vi "update fuel array.vi"(8 "Decrement fuel?":bool, 9 "Game Parameters":T3, 10 "step count":i32, 11 "Arrays and values":T1={"Score Array"=[], "Lowest high score"=0.0, "Score"=0.0, "Ceiling"=0.0, "Floor"=0.0, "Ceiling Array"=[], "Floor array"=[], "Helicopter height"=0.0, "Helicopter array"=[], "Fuel"=0.0, "Fuel array"=[], "fuel counter"=0, "obstacle counter"=0, "Obstacle array"=[], "helicopter v_0"=0.0, "helicopter a_0"=0.0, "Obstacle height"=300.0}) -> (2 "Fuel (L)":dbl(knob)=150.0 scale=0.0..300.0, 3 "Arrays and Heights":T1={"Score Array"=[], "Lowest high score"=0.0, "Score"=0.0, "Ceiling"=0.0, "Floor"=0.0, "Ceiling Array"=[], "Floor array"=[], "Helicopter height"=0.0, "Helicopter array"=[], "Fuel"=300.0, "Fuel array"=[], "fuel counter"=0, "obstacle counter"=0, "Obstacle array"=[], "helicopter v_0"=0.0, "helicopter a_0"=0.0, "Obstacle height"=300.0})   [LabVIEW 2017]
uses:
  controls/arrays and heights.ctl
  controls/scores.ctl
  controls/game parameters.ctl
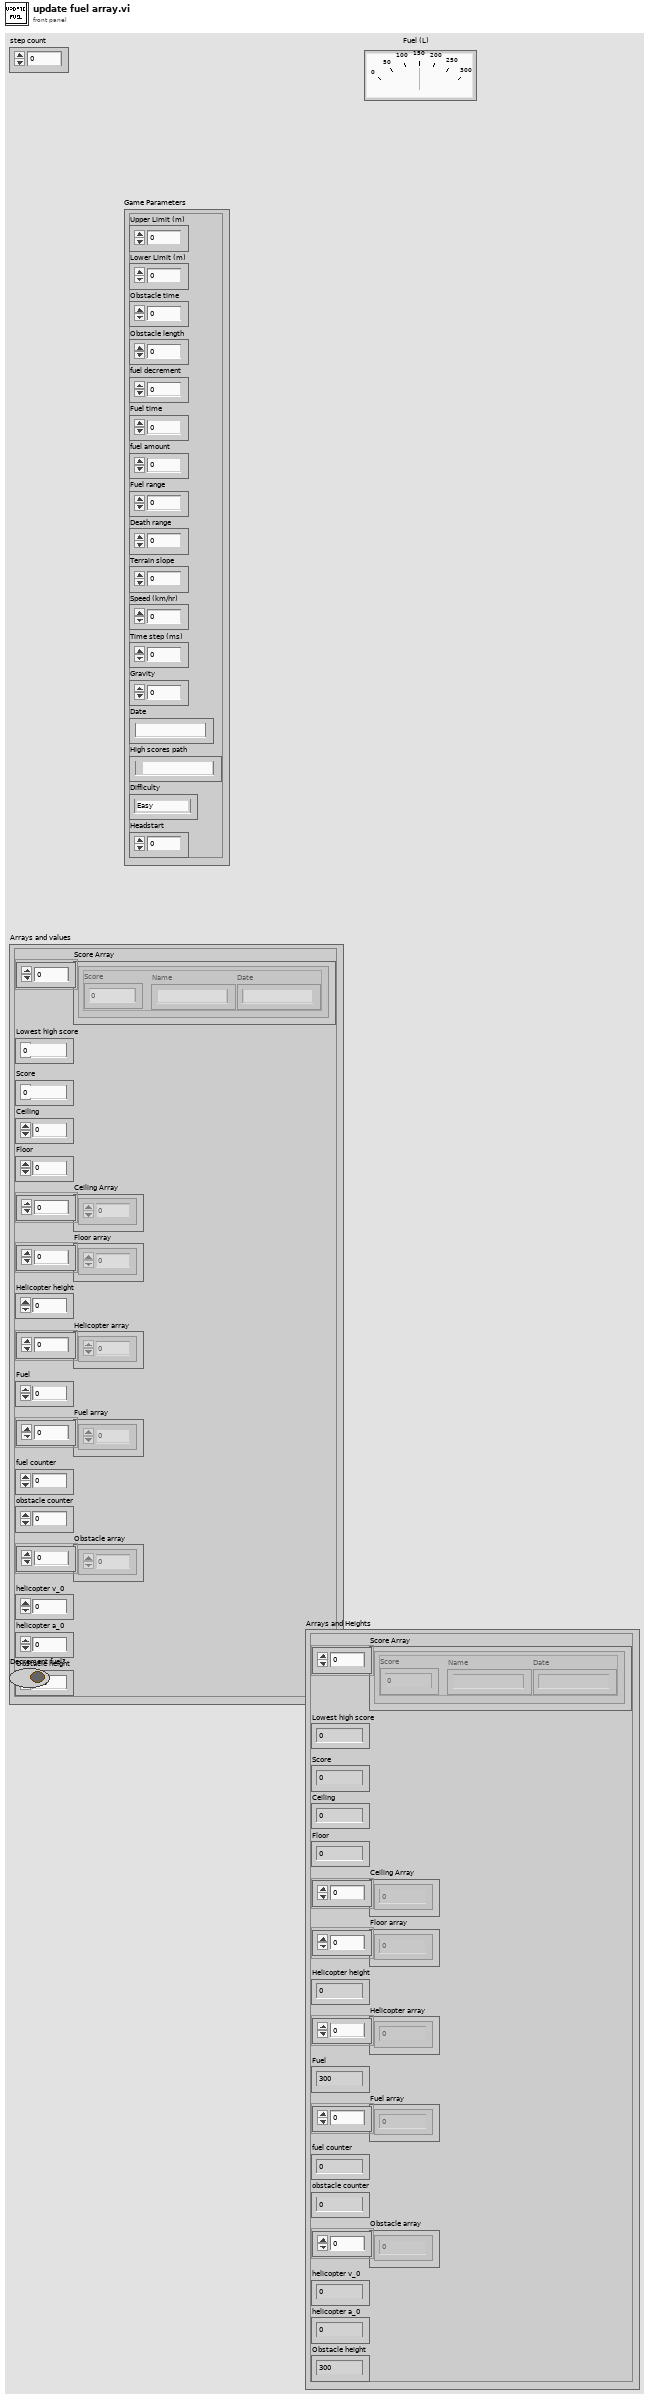
[diagram p1: front panel]
types:
  T1 = typedef "arrays and heights.ctl" = cluster{"Score Array":T2[], "Lowest high score":dbl, "Score":dbl, "Ceiling":dbl, "Floor":dbl, "Ceiling Array":dbl[], "Floor array":dbl[], "Helicopter height":dbl, "Helicopter array":dbl[], "Fuel":dbl, "Fuel array":dbl[], "fuel counter":i32, "obstacle counter":i32, "Obstacle array":dbl[], "helicopter v_0":dbl, "helicopter a_0":dbl, "Obstacle height":dbl}
  T2 = typedef "scores.ctl" = cluster{"Score":dbl, "Name":string, "Date":string}
  T3 = typedef "game parameters.ctl" = cluster{"Upper Limit (m)":dbl, "Lower Limit (m)":dbl, "Obstacle time":dbl, "Obstacle length":dbl, "fuel decrement":dbl, "Fuel time":dbl, "fuel amount":dbl, "Fuel range":i32, "Death range":i32, "Terrain slope":dbl, "Speed (km/hr)":dbl, "Time step (ms)":u32, "Gravity":dbl, "Date":string, "High scores path":path, "Difficulty":enum16{"Easy", "Normal", "Hard"}, "Headstart":u32}
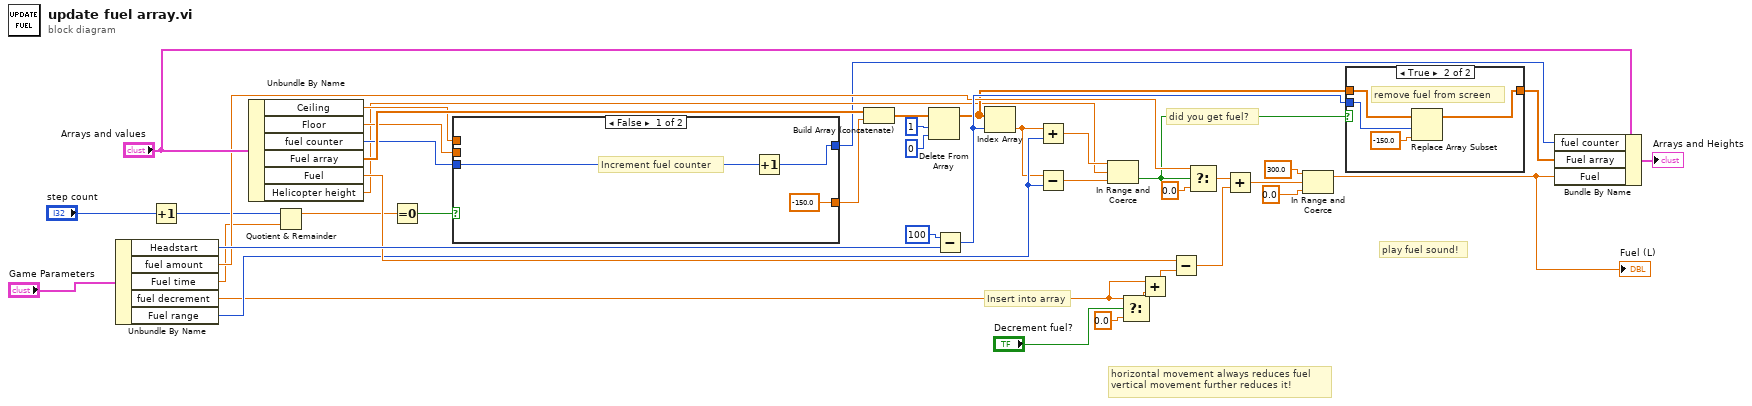
[diagram p0: block diagram]
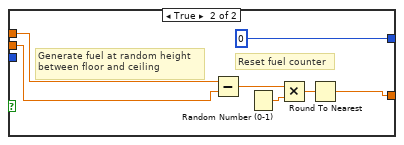
[diagram p3: hidden frame]
diagram:
  # "play fuel sound!"
  # "horizontal movement always reduces fuel\nvertical movement further reduces it!"
  # "did you get fuel?"
  # "Insert into array"
  n1 = Unbundle By Name("Game Parameters") -> ("Headstart"=w41:u32, "fuel amount"=w35:dbl, "Fuel time"=w3:dbl, "fuel decrement"=w1:dbl, "Fuel range"=w33:i32)
  n2 = Increment(x="step count") -> (x+1=w28:i32)
  n3 = Unbundle By Name("Arrays and values") -> ("Ceiling"=w30:dbl, "Floor"=w31:dbl, "fuel counter"=w32:i32, "Fuel array"=w36:dbl[], "Fuel"=w39:dbl, "Helicopter height"=w7:dbl)
  n4 = Quotient & Remainder(x=w28, y=w3) -> (x-y*floor(x/y)=w12:dbl)  [unwired: 1 out]
  n5 = Equal To 0?(x=w12) -> (x = 0?=w13:bool)
  n6 = case shown="False" w13 {
    tunnel: [-150.0 w50] -> w26
    tunnel: w32 -> [w45 _]
    tunnel: [w44 0] -> w6
    tunnel: w30 -> [_ w48]
    tunnel: w31 -> [_ w49]
    frame False {
      # "Increment fuel counter"
      n7 = Increment(x=w45) -> (x+1=w44:i32)
    }
    frame True {
      # "Reset fuel counter"
      # "Generate fuel at random height\nbetween floor and ceiling"
      n8 = Subtract(x=w48, y=w49) -> (x-y=w47:dbl)
      n9 = Random Number (0-1)() -> (number: 0 to 1=w52:dbl)
      n10 = Multiply(x=w47, y=w52) -> (x*y=w46:dbl)
      n11 = Round To Nearest(number=w46) -> (nearest integer value=w50:dbl)
    }
  }
  n12 = Build Array (concatenate)(w36, w26) -> (w14:dbl[])
  n13 = Delete From Array(array=w14, length=1, index=0) -> (array with subset deleted=w23:dbl[])  [unwired: 1 out]
  n14 = Subtract(x=u32 100, y=w41) -> (x-y=w42:u32)
  n15 = Index Array(array=w23, index=w42) -> (element=w19:dbl)
  n16 = Add(x=w19, y=w33) -> (x+y=w17:dbl)
  n17 = Subtract(x=w19, y=w33) -> (x-y=w18:dbl)
  n18 = In Range and Coerce(upper limit=w17, x=w7, lower limit=w18) -> (In Range?=w21:bool)  [unwired: 1 out]
  n19 = Select(t=w1, s="Decrement fuel?", f=0.0) -> (s? t:f=w9:dbl)
  n20 = Add(x=w1, y=w9) -> (x+y=w2:dbl)
  n21 = Subtract(x=w39, y=w2) -> (x-y=w11:dbl)
  n22 = Select(t=w35, s=w21, f=0.0) -> (s? t:f=w22:dbl)
  n23 = Add(x=w22, y=w11) -> (x+y=w24:dbl)
  n24 = In Range and Coerce(upper limit=300.0, x=w24, lower limit=0.0) -> (coerced(x)=w4:dbl)  [unwired: 1 out]
  "Fuel (L)" <- w4
  n25 = case shown="True" w21 {
    tunnel: w42 -> [_ w55]
    tunnel: w23 -> [w53 w57]
    tunnel: [w53 w56] -> w38
    frame False {
    }
    frame True {
      # "remove fuel from screen"
      n26 = Replace Array Subset(array=w57, new element=-150.0 ("new element/subarray"), index=w55) -> (w56:dbl[])
    }
  }
  n27 = Bundle By Name(cluster="Arrays and values", "fuel counter"=w6, "Fuel array"=w38, "Fuel"=w4) -> (→"Arrays and Heights":T1)
